vi "Histogram Window Specific Actions.vi"(6 "Top Menu":string, 7 "Histogram Graph Refnum":refnum<vi>, 8 "Error In":errorcluster, 9 "Menu Item Tag":string, 10 "Data in":variant, 11 "Histogram Window Internal Variables in":T1) -> (0 "Error Out":errorcluster, 3 "Histogram Window Internal Variables out":T1)   [LabVIEW 2019, in "Histogram Window.lvlib"]
uses:
  Histogram Window.lvlib
  Histogram Window Internal Variables.ctl
  Plot Histogram.ctl
  Graphs/Plot Style 3.ctl
  Variant/Variant to Data/Variant to Data.lvlib
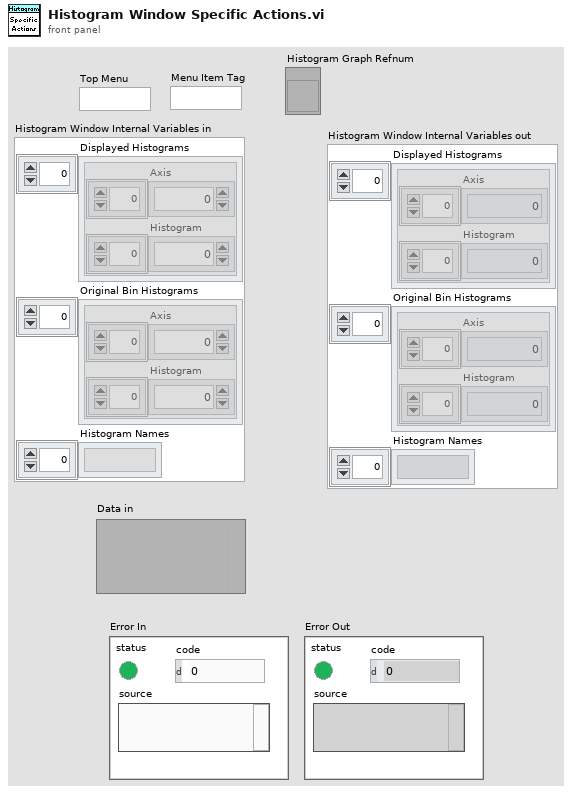
[diagram p1: front panel]
types:
  T1 = typedef "Histogram Window.lvlib/Histogram Window Internal Variables.ctl" = cluster{"Displayed Histograms":cluster{"Axis":dbl[], "Histogram":dbl[]}[], "Original Bin Histograms":cluster{"Axis":dbl[], "Histogram":dbl[]}[], "Histogram Names":string[]}
  T2 = typedef "Histogram Window.lvlib/Plot Histogram.ctl" = cluster{"Plot Name":string, "Histogram":cluster{"Axis":dbl[], "Histogram":dbl[]}, "Plot Style":T3}
  T3 = typedef "Plot Style 3.ctl" = cluster{"Plot Style":enum16{"unchanged", "Line", "Symbol", "Line + Symbol", "Histogram", "Histogram + Symbol"}, "Histogram Type":enum16{"unchanged", "Left Bound", "Center", "Right Bound"}, "Line Tickness":enum16{"unchanged", "Thin", "1 pixel", "2 pixel", "3 pixel", "4 pixel", "5 pixel"}, "Line Style":enum16{"unchanged", "Plain", "Long Dash", "Short Dash", "Long-Short Dash", "Long-Short-Short Dash"}, "Point Style":enum16{"unchanged", "None", "Empty Circle", "Filled Circle", "Thick Circle", "Dotted Circle", "Empty Square", "Filled Square", "Thick Square", "Dotted Square", "Small Filled Square", "Dot", "Cross", "Tiny Cross", "Large X", "Small x", "Diamond", "Small Empty Square"}, "Line Color":u32, "Point Color":u32, "Anti-aliased":bool, "Line Color Chooser":enum16{"unchanged", "Color Box", "Color List"}, "Point Color Chooser":enum16{"unchanged", "Color Box", "Color List"}, "Line Color List":string, "Point Color List":string}
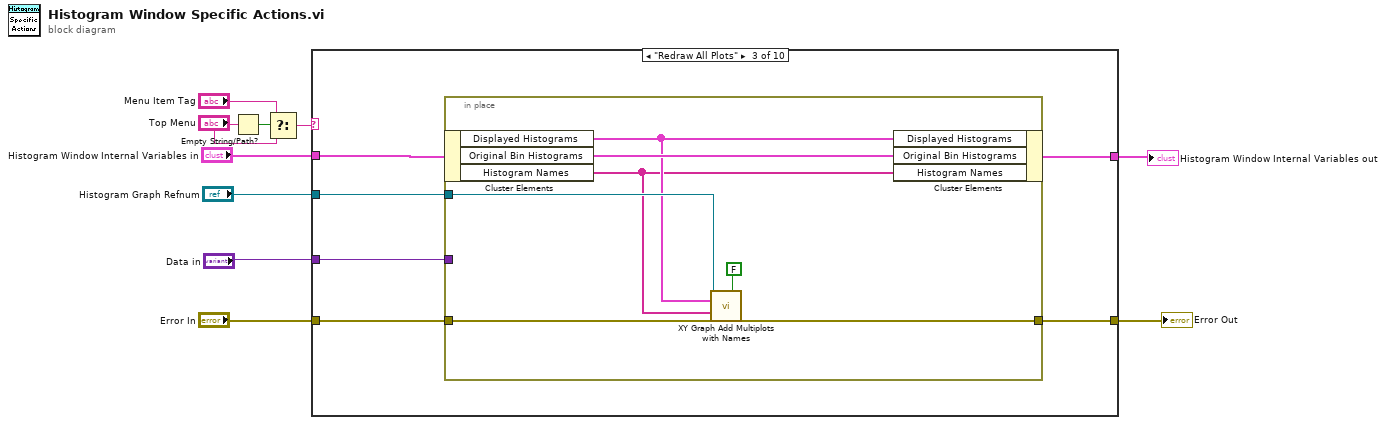
[diagram p0: block diagram]
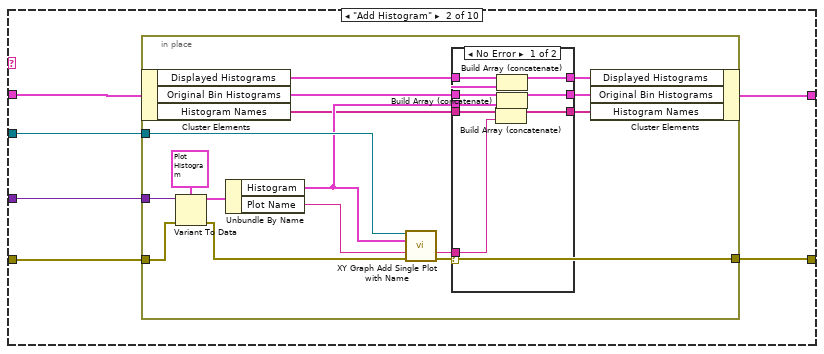
[diagram p3: hidden frame]
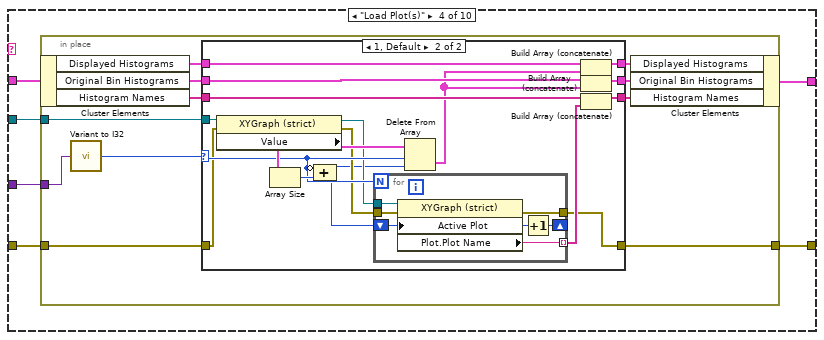
[diagram p5: hidden frame]
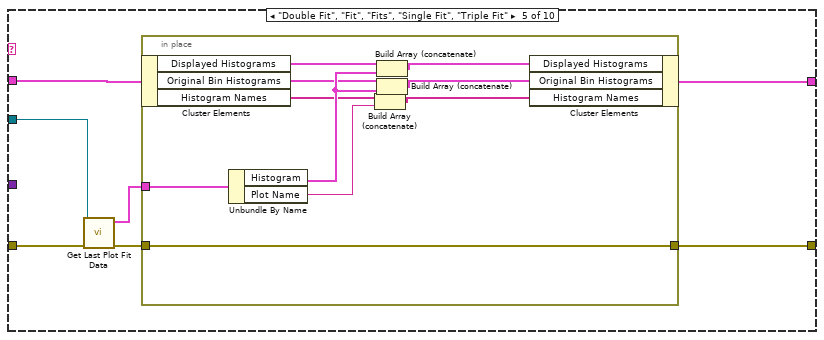
[diagram p7: hidden frame]
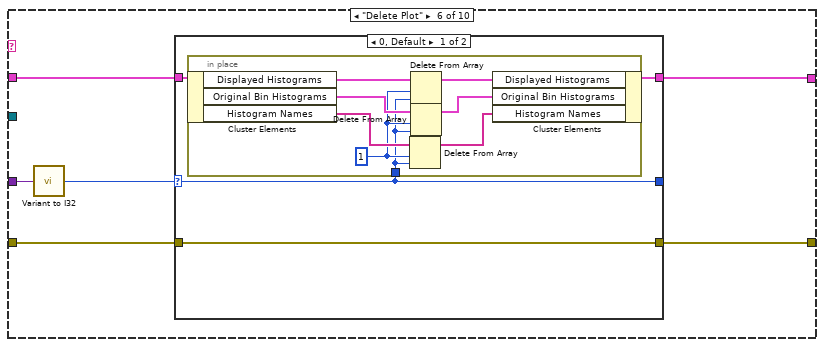
[diagram p8: hidden frame]
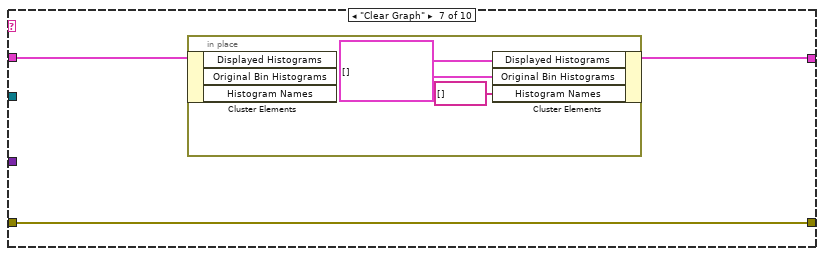
[diagram p10: hidden frame]
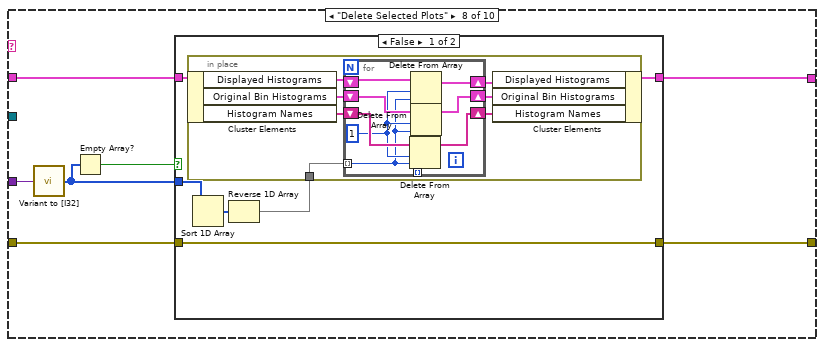
[diagram p11: hidden frame]
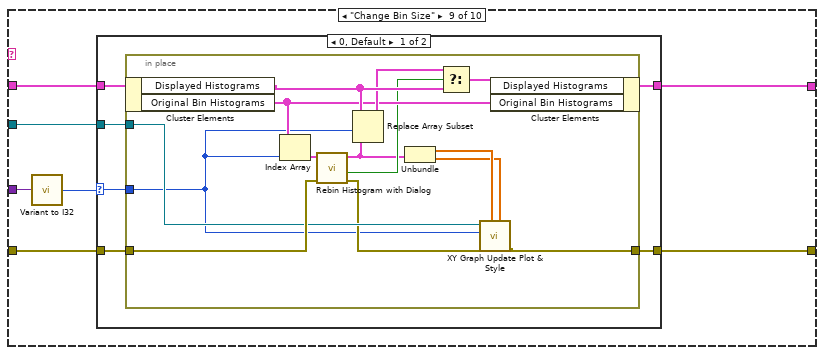
[diagram p13: hidden frame]
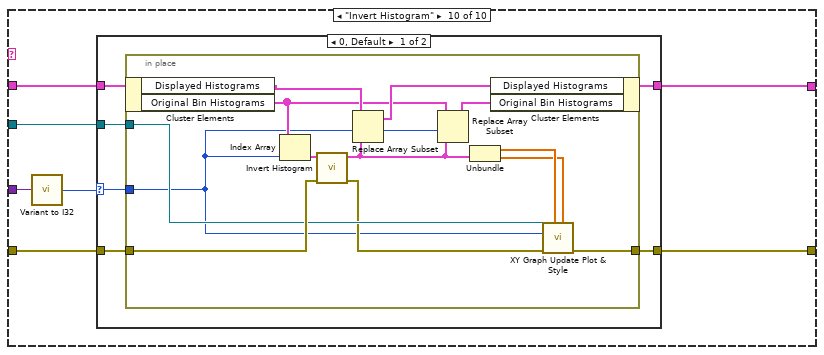
[diagram p15: hidden frame]
diagram:
  n1 = Empty String/Path?(string/path="Top Menu") -> (empty?=w4:bool)
  n2 = Select(t="Menu Item Tag", s=w4, f="Top Menu") -> (s? t:f=w2:string)
  n3 = case shown="\"Redraw All Plots\"" w2 {
    tunnel: "Histogram Window Internal Variables in" -> [w12 w17 w50 w63 w109 w125 w143 w152 w180 w209]
    tunnel: [w12 w16 w49 w62 w108 w122 w142 w150 w179 w208] -> w9
    tunnel: "Data in" -> [_ w18 w51 w64 _ w124 _ w151 w182 w211]
    tunnel: "Error In" -> [w11 w15 w48 w61 w104 w121 w141 w149 w178 w207]
    tunnel: [w11 w14 w46 w59 w103 w120 w141 w148 w177 w206] -> w6
    tunnel: "Histogram Graph Refnum" -> [_ w13 w47 w60 w105 _ _ _ w176 w205]
    frame "", Default {
    }
    frame "Add Histogram" {
      n4 = in-place {
        in-place-border: w18 -> [w31]
        in-place-border: w15 -> [w26]
        in-place-border: [w19] -> w14
        in-place-border: w13 -> [w24]
        n5 = in-place-cluster #1(w17) -> ("Displayed Histograms"=w30:cluster{"Axis":dbl[], "Histogram":dbl[]}[], "Original Bin Histograms"=w28:cluster{"Axis":dbl[], "Histogram":dbl[]}[], "Histogram Names"=w21:string[])
        n6 = Variant To Data(error in=w26, type=T2 {"Plot Name"="", "Histogram"={"Axis"=[], "Histogram"=[]}, "Plot Style"={"Plot Style"=enum."Histogram + Symbol", "Histogram Type"=enum."Right Bound", "Line Tickness"=enum."unchanged", "Line Style"=enum."unchanged", "Point Style"=enum."unchanged", "Line Color"=0, "Point Color"=0, "Anti-aliased"=FALSE, "Line Color Chooser"=enum."unchanged", "Point Color Chooser"=enum."unchanged", "Line Color List"="", "Point Color List"=""}} ("output cluster"), Variant=w31) -> (data=w34:T2, error out=w25:errorcluster)
        n7 = Unbundle By Name(w34) -> ("Histogram"=w23:cluster{"Axis":dbl[], "Histogram":dbl[]}, "Plot Name"=w33:string)
        n8 = call "XY Graph Add Single Plot with Name.vi"("XYGraph Ref in"=w24, "Plot"=w23, "Plot Name (\"Plot\")"=w33, "error in (no error)"=w25) -> ("Plot Name"=w20:string, "error out"=w19:errorcluster)  [unwired: 8 in, 2 out]
        n9 = case shown="No Error" w19 {
          tunnel: w30 -> [w42 w45]
          tunnel: [w41 w45] -> w29
          tunnel: w28 -> [w40 w44]
          tunnel: [w39 w44] -> w27
          tunnel: w23 -> [w38 _]
          tunnel: [w37 w43] -> w22
          tunnel: w21 -> [w36 w43]
          tunnel: w20 -> [w35 _]
          frame No Error {
            n10 = Build Array (concatenate)(w36, w35) -> (w37:string[])
            n11 = Build Array (concatenate)(w42, w38) -> (w41:cluster{"Axis":dbl[], "Histogram":dbl[]}[])
            n12 = Build Array (concatenate)(w40, w38) -> (w39:cluster{"Axis":dbl[], "Histogram":dbl[]}[])
          }
          frame Error {
          }
        }
        n13 = in-place-cluster #1("Displayed Histograms"=w29, "Original Bin Histograms"=w27, "Histogram Names"=w22) -> (w16:T1)
      }
    }
    frame "Redraw All Plots" {
      n14 = in-place {
        in-place-border: w51 -> [_]
        in-place-border: w48 -> [w56]
        in-place-border: w47 -> [w57]
        in-place-border: [w55] -> w46
        n15 = in-place-cluster #2(w50) -> ("Displayed Histograms"=w54:cluster{"Axis":dbl[], "Histogram":dbl[]}[], "Original Bin Histograms"=w58:cluster{"Axis":dbl[], "Histogram":dbl[]}[], "Histogram Names"=w53:string[])
        n16 = call "XY Graph Add Multiplots with Names.vi"("XYGraph in"=w57, "Keep Existing Plots (T)"=FALSE, "Array of Plots"=w54, "Array of Plot Names (\"Plot\")"=w53, "error in (no error)"=w56) -> ("error out"=w55:errorcluster)  [unwired: 6 in, 4 out]
        n17 = in-place-cluster #2("Displayed Histograms"=w54, "Original Bin Histograms"=w58, "Histogram Names"=w53) -> (w49:T1)
      }
    }
    frame "Load Plot(s)" {
      n18 = in-place {
        in-place-border: w64 -> [w68]
        in-place-border: w61 -> [w67]
        in-place-border: w60 -> [w66]
        in-place-border: [w65] -> w59
        n19 = in-place-cluster #3(w63) -> ("Displayed Histograms"=w75:cluster{"Axis":dbl[], "Histogram":dbl[]}[], "Original Bin Histograms"=w74:cluster{"Axis":dbl[], "Histogram":dbl[]}[], "Histogram Names"=w70:string[])
        n20 = call "Variant to I32.vi"("Variant"=w68) -> ("Value"=w73:i32)  [unwired: 8 in]
        n21 = case shown="1, Default" w73 {
          selector: w73 -> [_ w87]
          tunnel: w75 -> [w79 w96]
          tunnel: w74 -> [w78 w95]
          tunnel: [w79 w90] -> w72
          tunnel: [w78 w89] -> w71
          tunnel: w70 -> [w77 w94]
          tunnel: [w77 w83] -> w69
          tunnel: w67 -> [w76 w81]
          tunnel: w66 -> [_ w93]
          tunnel: [w76 w80] -> w65
          frame 0 {
          }
          frame 1, Default {
            n22 = property class="XYGraph (strict)"(reference=w93, error in=w81) -> (reference out=w86:refnum<vi>, error out=w85:errorcluster, "Value"=w92:cluster{"Axis":dbl[], "Histogram":dbl[]}[])
            n23 = Array Size(array=w92) -> (size(s)=w91:i32)
            n24 = Compound Arithmetic op=ADD(invert w87, w91) -> (w84:i32)
            n25 = for {
              N: w87 -> [_]
              tunnel: w86 -> [w102]
              tunnel: w85 -> [w101]
              shift-right: [w99] -> _
              shift-left: w84 -> [w100]
              tunnel: [w98] -> w82 mode=indexing
              tunnel: [w97] -> w80
              n26 = property class="XYGraph (strict)"(reference=w102, error in=w101, "Active Plot"=w100) -> (error out=w97:errorcluster, "Plot.Plot Name"=w98:string)  [unwired: 1 out]
              n27 = Increment(x=w100) -> (x+1=w99:i32)
            }
            n28 = Delete From Array(array=w92, length=w87, index=w84) -> (deleted portion=w88:cluster{"Axis":dbl[], "Histogram":dbl[]}[])  [unwired: 1 out]
            n29 = Build Array (concatenate)(w96, w88) -> (w90:cluster{"Axis":dbl[], "Histogram":dbl[]}[])
            n30 = Build Array (concatenate)(w95, w88) -> (w89:cluster{"Axis":dbl[], "Histogram":dbl[]}[])
            n31 = Build Array (concatenate)(w94, w82) -> (w83:string[])
          }
        }
        n32 = in-place-cluster #3("Displayed Histograms"=w72, "Original Bin Histograms"=w71, "Histogram Names"=w69) -> (w62:T1)
      }
    }
    frame "Double Fit", "Fit", "Fits", "Single Fit", "Triple Fit" {
      n33 = call "Get Last Plot Fit Data.vi"("error in (no error)"=w104, "XYGraph in"=w105) -> ("error out"=w107:errorcluster, "Last Fit Data"=w106:T2)  [unwired: 8 in]
      n34 = in-place {
        in-place-border: w107 -> [w110]
        in-place-border: w106 -> [w114]
        in-place-border: [w110] -> w103
        n35 = in-place-cluster #4(w109) -> ("Displayed Histograms"=w118:cluster{"Axis":dbl[], "Histogram":dbl[]}[], "Original Bin Histograms"=w116:cluster{"Axis":dbl[], "Histogram":dbl[]}[], "Histogram Names"=w113:string[])
        n36 = Unbundle By Name(w114) -> ("Histogram"=w119:cluster{"Axis":dbl[], "Histogram":dbl[]}, "Plot Name"=w112:string)
        n37 = Build Array (concatenate)(w113, w112) -> (w111:string[])
        n38 = Build Array (concatenate)(w118, w119) -> (w117:cluster{"Axis":dbl[], "Histogram":dbl[]}[])
        n39 = Build Array (concatenate)(w116, w119) -> (w115:cluster{"Axis":dbl[], "Histogram":dbl[]}[])
        n40 = in-place-cluster #4("Displayed Histograms"=w117, "Original Bin Histograms"=w115, "Histogram Names"=w111) -> (w108:T1)
      }
    }
    frame "Delete Plot" {
      n41 = call "Variant to I32.vi"("Variant"=w124) -> ("Value"=w123:i32)  [unwired: 8 in]
      n42 = case shown="0, Default" w123 {
        selector: w123 -> [w126 w138]
        tunnel: w125 -> [w129 w140]
        tunnel: [w128 w140] -> w122
        tunnel: [w127 w139] -> w120
        tunnel: w121 -> [w127 w139]
        tunnel: [w126 w138] -> _
        frame 0, Default {
          n43 = in-place {
            in-place-border: w126 -> [w130]
            w131 = 1 ("length")
            n44 = in-place-cluster #5(w129) -> ("Displayed Histograms"=w137:cluster{"Axis":dbl[], "Histogram":dbl[]}[], "Original Bin Histograms"=w135:cluster{"Axis":dbl[], "Histogram":dbl[]}[], "Histogram Names"=w133:string[])
            n45 = Delete From Array(array=w133, length=w131, index=w130) -> (array with subset deleted=w132:string[])  [unwired: 1 out]
            n46 = Delete From Array(array=w137, length=w131, index=w130) -> (array with subset deleted=w136:cluster{"Axis":dbl[], "Histogram":dbl[]}[])  [unwired: 1 out]
            n47 = Delete From Array(array=w135, length=w131, index=w130) -> (array with subset deleted=w134:cluster{"Axis":dbl[], "Histogram":dbl[]}[])  [unwired: 1 out]
            n48 = in-place-cluster #5("Displayed Histograms"=w136, "Original Bin Histograms"=w134, "Histogram Names"=w132) -> (w128:T1)
          }
        }
        frame -1 {
        }
      }
    }
    frame "Clear Graph" {
      n49 = in-place {
        w145 = cluster{"Axis":dbl[], "Histogram":dbl[]}[] [] ("Displayed Histograms")
        n50 = in-place-cluster #6(w143) -> ()  [unwired: 3 out]
        n51 = in-place-cluster #6("Displayed Histograms"=w145, "Original Bin Histograms"=w145, "Histogram Names"=string[] []) -> (w142:T1)
      }
    }
    frame "Delete Selected Plots" {
      n52 = call "Variant to [I32].vi"("Variant"=w151) -> ("Value"=w146:i32[])  [unwired: 8 in]
      n53 = Empty Array?(array=w146) -> (empty?=w147:bool)
      n54 = case shown="False" w147 {
        tunnel: w152 -> [w158 w175]
        tunnel: [w157 w175] -> w150
        tunnel: [w156 w174] -> w148
        tunnel: w149 -> [w156 w174]
        tunnel: w146 -> [w153 _]
        frame False {
          n55 = Sort 1D Array(array=w153) -> (sorted array=w155:i32[])
          n56 = Reverse 1D Array(array=w155) -> (reversed array=w154:i32[])
          n57 = in-place {
            in-place-border: w154 -> [w160]
            n58 = in-place-cluster #7(w158) -> ("Displayed Histograms"=w165:cluster{"Axis":dbl[], "Histogram":dbl[]}[], "Original Bin Histograms"=w164:cluster{"Axis":dbl[], "Histogram":dbl[]}[], "Histogram Names"=w162:string[])
            n59 = for {
              tunnel: [w167] -> _ mode=indexing
              tunnel: w160 -> [w167] mode=indexing
              shift-right: [w166] -> w159
              shift-left: w165 -> [w173]
              shift-right: [w171] -> w163
              shift-left: w164 -> [w172]
              shift-right: [w169] -> w161
              shift-left: w162 -> [w170]
              w168 = 1 ("length")
              n60 = Delete From Array(array=w170, length=w168, index=w167) -> (array with subset deleted=w169:string[])  [unwired: 1 out]
              n61 = Delete From Array(array=w173, length=w168, index=w167) -> (array with subset deleted=w166:cluster{"Axis":dbl[], "Histogram":dbl[]}[])  [unwired: 1 out]
              n62 = Delete From Array(array=w172, length=w168, index=w167) -> (array with subset deleted=w171:cluster{"Axis":dbl[], "Histogram":dbl[]}[])  [unwired: 1 out]
            }
            n63 = in-place-cluster #7("Displayed Histograms"=w159, "Original Bin Histograms"=w163, "Histogram Names"=w161) -> (w157:T1)
          }
        }
        frame True {
        }
      }
    }
    frame "Change Bin Size" {
      n64 = call "Variant to I32.vi"("Variant"=w182) -> ("Value"=w181:i32)  [unwired: 8 in]
      n65 = case shown="0, Default" w181 {
        selector: w181 -> [w187 _]
        tunnel: w180 -> [w188 w204]
        tunnel: [w185 w204] -> w179
        tunnel: w178 -> [w186 w203]
        tunnel: [w184 w203] -> w177
        tunnel: w176 -> [w183 _]
        frame 0, Default {
          n66 = in-place {
            in-place-border: w187 -> [w192]
            in-place-border: w186 -> [w201]
            in-place-border: [w193] -> w184
            in-place-border: w183 -> [w195]
            n67 = in-place-cluster #8(w188) -> ("Displayed Histograms"=w199:cluster{"Axis":dbl[], "Histogram":dbl[]}[], "Original Bin Histograms"=w197:cluster{"Axis":dbl[], "Histogram":dbl[]}[])
            n68 = Index Array(array=w197, index=w192) -> (element=w202:cluster{"Axis":dbl[], "Histogram":dbl[]})
            n69 = call "Rebin Histogram with Dialog.vi"("error in (no error)"=w201, "Original Bin Histogram"=w202) -> ("error out"=w194:errorcluster, "OK?"=w196:bool, "Rebinned Histogram"=w191:cluster{"Axis":dbl[], "Histogram":dbl[]})  [unwired: 7 in]
            n70 = Replace Array Subset(array=w199, new element=w191, index=w192) -> (w198:cluster{"Axis":dbl[], "Histogram":dbl[]}[])
            n71 = Unbundle(w191) -> ("Axis"=w190:dbl[], "Histogram"=w189:dbl[])
            n72 = Select(t=w198, s=w196, f=w199) -> (s? t:f=w200:cluster{"Axis":dbl[], "Histogram":dbl[]}[])
            n73 = call "XY Graph Update Plot & Style.vi"("Y Array"=w189, "X Array"=w190, "Error In"=w194, "Plot Idx"=w192, "XY Graph refnum"=w195) -> ("Error Out"=w193:errorcluster)  [unwired: 4 in, 2 out]
            n74 = in-place-cluster #8("Displayed Histograms"=w200, "Original Bin Histograms"=w197) -> (w185:T1)
          }
        }
        frame -1 {
        }
      }
    }
    frame "Invert Histogram" {
      n75 = call "Variant to I32.vi"("Variant"=w211) -> ("Value"=w210:i32)  [unwired: 8 in]
      n76 = case shown="0, Default" w210 {
        selector: w210 -> [w216 _]
        tunnel: w209 -> [w217 w232]
        tunnel: [w214 w232] -> w208
        tunnel: w207 -> [w215 w231]
        tunnel: [w213 w231] -> w206
        tunnel: w205 -> [w212 _]
        frame 0, Default {
          n77 = in-place {
            in-place-border: w216 -> [w218]
            in-place-border: w215 -> [w229]
            in-place-border: [w219] -> w213
            in-place-border: w212 -> [w221]
            n78 = in-place-cluster #9(w217) -> ("Displayed Histograms"=w228:cluster{"Axis":dbl[], "Histogram":dbl[]}[], "Original Bin Histograms"=w226:cluster{"Axis":dbl[], "Histogram":dbl[]}[])
            n79 = Index Array(array=w226, index=w218) -> (element=w230:cluster{"Axis":dbl[], "Histogram":dbl[]})
            n80 = call "Invert Histogram.vi"("error in (no error)"=w229, "Histogram"=w230) -> ("error out"=w220:errorcluster, "Inverted Histogram"=w222:cluster{"Axis":dbl[], "Histogram":dbl[]})  [unwired: 8 in]
            n81 = Replace Array Subset(array=w228, new element=w222, index=w218) -> (w227:cluster{"Axis":dbl[], "Histogram":dbl[]}[])
            n82 = Replace Array Subset(array=w226, new element=w222, index=w218) -> (w225:cluster{"Axis":dbl[], "Histogram":dbl[]}[])
            n83 = Unbundle(w222) -> ("Axis"=w224:dbl[], "Histogram"=w223:dbl[])
            n84 = in-place-cluster #9("Displayed Histograms"=w227, "Original Bin Histograms"=w225) -> (w214:T1)
            n85 = call "XY Graph Update Plot & Style.vi"("Y Array"=w223, "X Array"=w224, "Error In"=w220, "Plot Idx"=w218, "XY Graph refnum"=w221) -> ("Error Out"=w219:errorcluster)  [unwired: 4 in, 2 out]
          }
        }
        frame -1 {
        }
      }
    }
  }
  "Histogram Window Internal Variables out" <- w9
  "Error Out" <- w6
